vi "rad_ExtractNestedImage.vi"(8 "error in":errorcluster, 10 "TempFolderPath":path, 11 "image file path":path) -> (0 "error out":errorcluster, 2 "Unzipped files":path[](array[path]), 3 "NestedImagePath":path)   [LabVIEW 2013]
uses:
  <vilib>/zip/NI_Unzip.lvlib
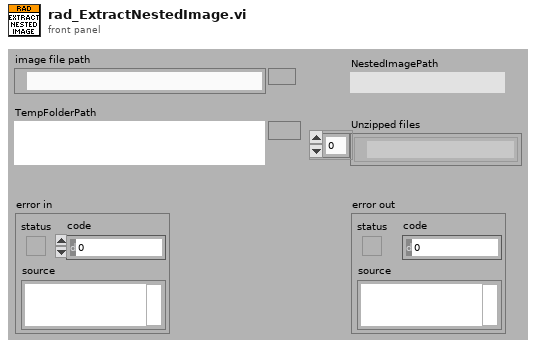
[diagram p1: front panel]
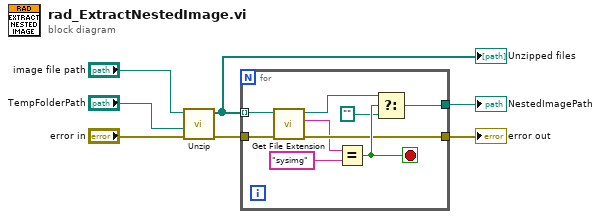
[diagram p0: block diagram]
diagram:
  n1 = call <vilib>:"Unzip.vi"("error in (no error)"="error in", "Target directory (same as Zip file if empty)"="TempFolderPath", "Zip file"="image file path") -> ("error out"=w4:errorcluster, "Unzipped files"=w3:path[])  [unwired: 6 in, 1 out]
  "Unzipped files" <- w3
  n2 = for {
    tunnel: w3 -> [w9] mode=indexing
    tunnel: w4 -> [w15]
    tunnel: [w12] -> w2
    tunnel: [w11] -> w1
    stop <- w14 stop-if-true
    n3 = call <vilib>:"Get File Extension.vi"("error in (no error)"=w15, "file"=w9) -> ("error out"=w11:errorcluster, "lowercase file extension"=w10:string, "dup file"=w8:path)  [unwired: 6 in, 1 out]
    n4 = Equal?(x=w10, y="sysimg" ("string")) -> (x = y?=w14:bool)
    n5 = Select(t=w8, s=w14, f=path "") -> (s? t:f=w12:path)
  }
  "error out" <- w1
  "NestedImagePath" <- w2
